vi "MCLB Edit Cell.vi"(8 "error in (no error)":errorcluster, 11 "View in":refnum<class "MCListbox View.lvclass">) -> (0 "error out":errorcluster, 3 "View out":refnum<class "MCListbox View.lvclass">)   [LabVIEW 2013, in "SET Project Editor.lvlib" / "MCListbox View.lvclass"]
uses:
  MCListbox View.lvclass
  MCListbox View.lvclass/MCListbox View.ctl
  <vilib>/Utility/miscctls.llb/LVPositionTypeDef.ctl
  <vilib>/Utility/miscctls.llb/LVBoundsTypeDef.ctl
  Lib/Unicode/SET_Unicode Tools.lvlib
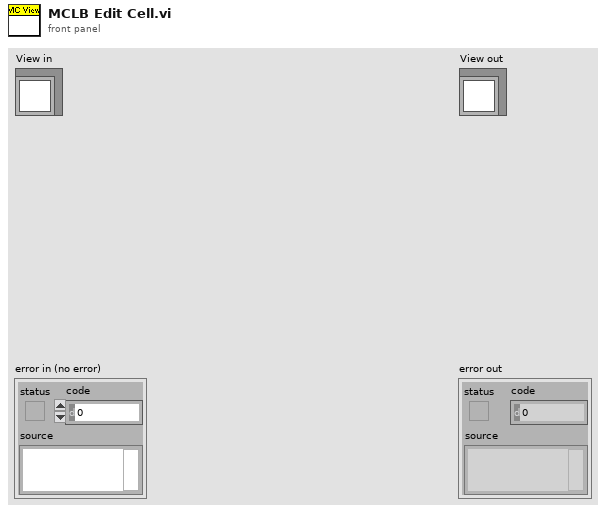
[diagram p1: front panel]
types:
  T1 = typedef "LVBoundsTypeDef.ctl" = cluster{"Width":u32, "Height":u32}
  T2 = typedef "LVPositionTypeDef.ctl" = cluster{"Left":i32, "Top":i32}
  T3 = typedef "LVRowAndColumnTypeDef.ctl" = cluster{"Row":i32, "Column":i32}
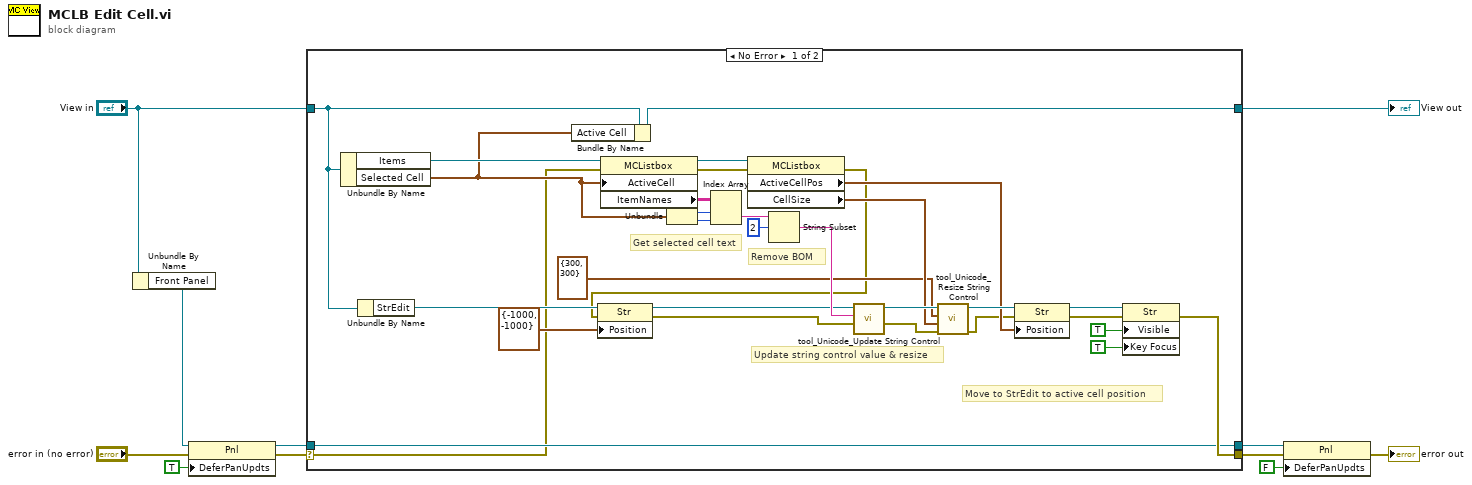
[diagram p0: block diagram]
diagram:
  n1 = Unbundle By Name("View in") -> ("Front Panel"=w9:refnum<vi>)
  n2 = property class="Pnl"(reference=w9, error in="error in (no error)", "DeferPanUpdts"=TRUE ("Defer Panel Updates")) -> (reference out=w5:refnum<vi>, error out=w7:errorcluster)
  n3 = case shown="No Error" w7 {
    selector: w7 -> [w13 w45]
    tunnel: [w17 w45] -> w1
    tunnel: [w14 w44] -> w11
    tunnel: "View in" -> [w15 w44]
    tunnel: w5 -> [w16 w43]
    tunnel: [w16 w43] -> w2
    frame No Error {
      # "Move to StrEdit to active cell position"
      # "Update string control value & resize"
      # "Get selected cell text"
      # "Remove BOM"
      n4 = Unbundle By Name(w15) -> ("Items"=w42:refnum<vi>, "Selected Cell"=w31:T3)
      n5 = Unbundle By Name(w15) -> ("StrEdit"=w27:refnum<vi>)
      n6 = Bundle By Name(cluster=w15, "Active Cell"=w31) -> (w14:refnum<class "MCListbox View.lvclass">)
      n7 = property class="MCListbox"(reference=w42, error in=w13, "ActiveCell"=w31) -> (reference out=w36:refnum<vi>, error out=w30:errorcluster, "ItemNames"=w39:string[][])
      n8 = Unbundle(w31) -> ("Row"=w38:i32, "Column"=w37:i32)
      n9 = Index Array(array=w39, index (row)=w38, index (col)=w37) -> (element=w40:string)
      n10 = property class="MCListbox"(reference=w36, error in=w30) -> (error out=w12:errorcluster, "ActiveCellPos"=w24:T2, "CellSize"=w29:T1)  [unwired: 1 out]
      n11 = property class="Str"(reference=w27, error in=w12, "Position"=T2 {"Left"=-1000, "Top"=-1000}) -> (reference out=w19:refnum<vi>, error out=w18:errorcluster)
      n12 = String Subset(string=w40, offset (0)=2) -> (substring=w35:string)  [unwired: 1 in]
      n13 = call "tool_Unicode_Update String Control.vi"("error in (no error)"=w18, "String (UTF-16)"=w35, "*StrControl in"=w19) -> ("error out"=w28:errorcluster, "*StrControl out"=w34:refnum<vi>)  [unwired: 7 in]
      n14 = call "tool_Unicode_Resize String Control.vi"("error in (no error)"=w28, "Min Size (10x10)"=w29, "Max Size (300x300)"=T1 {"Width"=300, "Height"=300}, "*StrControl in"=w34) -> ("error out"=w23:errorcluster, "*StrControl out"=w25:refnum<vi>)  [unwired: 6 in]
      n15 = property class="Str"(reference=w25, error in=w23, "Position"=w24) -> (reference out=w22:refnum<vi>, error out=w21:errorcluster)
      n16 = property class="Str"(reference=w22, error in=w21, "Visible"=TRUE, "Key Focus"=TRUE) -> (error out=w17:errorcluster)  [unwired: 1 out]
    }
    frame Error {
    }
  }
  "View out" <- w11
  n17 = property class="Pnl"(reference=w2, error in=w1, "DeferPanUpdts"=FALSE ("Defer Panel Updates")) -> (error out=→"error out":errorcluster)  [unwired: 1 out]
